vi "terminate.vi"(8 "error in (no error)":errorcluster, 11 "StageMG100204SutterMP285 in":refnum<class "StageMG100204SutterMP285.lvclass">=refnum) -> (0 "error out":errorcluster, 3 "StageMG100204SutterMP285 out":refnum<class "StageMG100204SutterMP285.lvclass">)   [LabVIEW 2010, in "StageMG100204SutterMP285.lvclass"]
doc: "The dynamic dispatch version of this VI terminates the plug-in object by releasing all of its resources."
uses:
  StageMG100204SutterMP285.lvclass
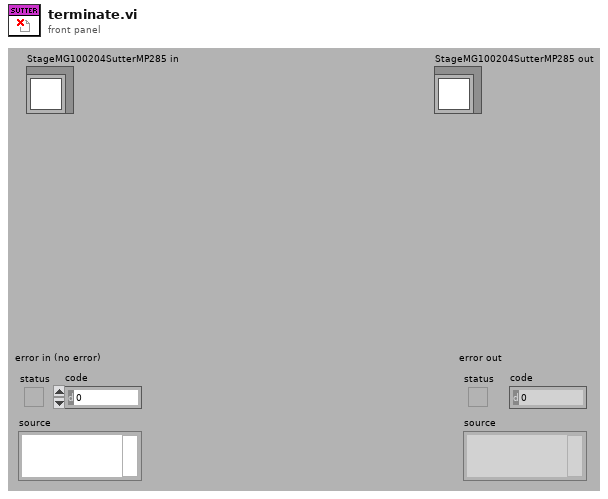
[diagram p1: front panel]
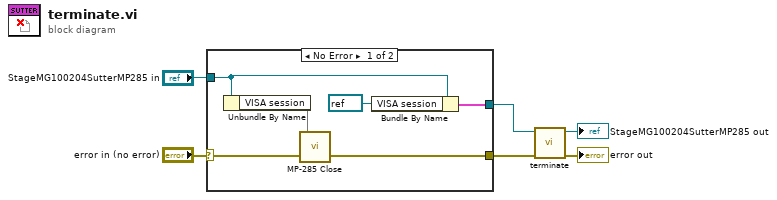
[diagram p0: block diagram]
diagram:
  n1 = case shown="No Error" "error in (no error)" {
    selector: "error in (no error)" -> [w12 w14]
    tunnel: [w11 w14] -> w5
    tunnel: "StageMG100204SutterMP285 in" -> [w9 w13]
    tunnel: [w8 w13] -> w4
    frame No Error {
      n2 = Unbundle By Name(w9) -> ("VISA session"=w10)
      n3 = call "MP-285 Close.vi"("error in (no error)"=w12, "VISA resource name"=w10) -> ("Output: Error cluster"=w11:errorcluster)  [unwired: 1 out]
      n4 = Bundle By Name(cluster=w9, "VISA session"=refnum<visa-resource-name> refnum) -> (w8:cluster{})
    }
    frame Error {
    }
  }
  n5 = call-parent "terminate.vi"("error in (no error)"=w5, "GenericPlugin in"=w4) -> ("error out"=→"error out":errorcluster, "GenericPlugin out"=→"StageMG100204SutterMP285 out":refnum<class "StageMG100204SutterMP285.lvclass">)  [unwired: 8 out]
